vi "SwissSPAD Live_Correct SS3 Gate Slippage [U16].vi"(8 "Error In":errorcluster, 11 "Array in":u16[][](array[numeric])) -> (0 "Error Out":errorcluster, 2 "Checkbox":bool, 3 "Array out":u16[][](array[numeric]))   [LabVIEW 2021, in "SwissSPAD Live.lvlib"]
uses:
  SwissSPAD Live.lvlib
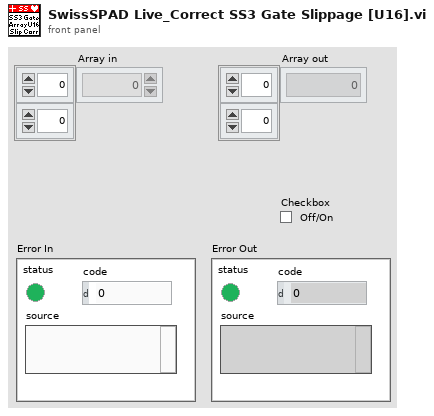
[diagram p1: front panel]
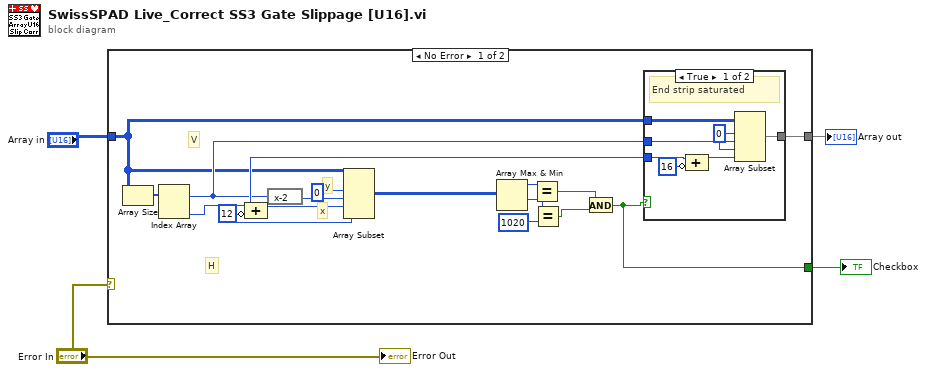
[diagram p0: block diagram]
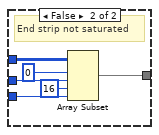
[diagram p2: hidden frame]
diagram:
  n1 = case shown="No Error" "Error In" {
    tunnel: [w16 _] -> w4
    tunnel: [w15 w34] -> w3
    tunnel: "Array in" -> [w14 w34]
    frame No Error {
      w13 = 12 ("value")
      # "H"
      # "V"
      # "x"
      # "y"
      n2 = Array Size(array=w14) -> (size(s)=w5:i32[])
      n3 = Index Array(array=w5) -> (element #1=w17:i32, element #2=w18:i32)  [unwired: 2 in]
      n4 = Compound Arithmetic op=ADD(w18, invert w13) -> (w12:i32)
      n5 = expression code="x-2"(w17) -> (w19:i32)
      n6 = Array Subset(array=w14, index (row)=0 ("length"), length (row)=w19, index (col)=w12, length (col)=w13) -> (w20:u16[][])
      n7 = Array Max & Min(array=w20) -> (max value=w7:u16, min value=w8:u16)  [unwired: 2 out]
      n8 = Equal?(x=w7, y=w8) -> (x = y?=w10:bool)
      n9 = Equal?(x=w8, y=u16 1020) -> (x = y?=w11:bool)
      n10 = And(x=w10, y=w11) -> (x .and. y?=w16:bool)
      n11 = case shown="True" w16 {
        tunnel: w14 -> [w27 w33]
        tunnel: w17 -> [w26 w32]
        tunnel: w18 -> [w23 w30]
        tunnel: [w24 w29] -> w15
        frame True {
          w25 = 0 ("index")
          # "End strip saturated"
          n12 = Compound Arithmetic op=ADD(w23, invert 16 ("value")) -> (w21:i32)
          n13 = Array Subset(array=w27, index (row)=w25, length (row)=w26, index (col)=w25, length (col)=w21) -> (w24:u16[][])
        }
        frame False {
          # "End strip not saturated"
          n14 = Array Subset(array=w33, index (row)=0 ("index"), length (row)=w32, index (col)=16 ("index"), length (col)=w30) -> (w29:u16[][])
        }
      }
    }
    frame Error {
    }
  }
  "Checkbox" <- w4
  "Array out" <- w3
  "Error Out" <- "Error In"
